vi "Get HSB.vi"(8 "error in (no error)":errorcluster caption="错误输入（无错误）", 11 "Color 输入":refnum<class "Color.lvclass"> caption="DNL_LabVIEW Object in") -> (0 "error out":errorcluster caption="错误输出", 2 "HSB":T1, 3 "Color 输出":refnum<class "Color.lvclass"> caption="DNL_LabVIEW Object out")   [LabVIEW 2012, in "Color.lvclass"]
uses:
  Color.lvclass
  HSB.ctl
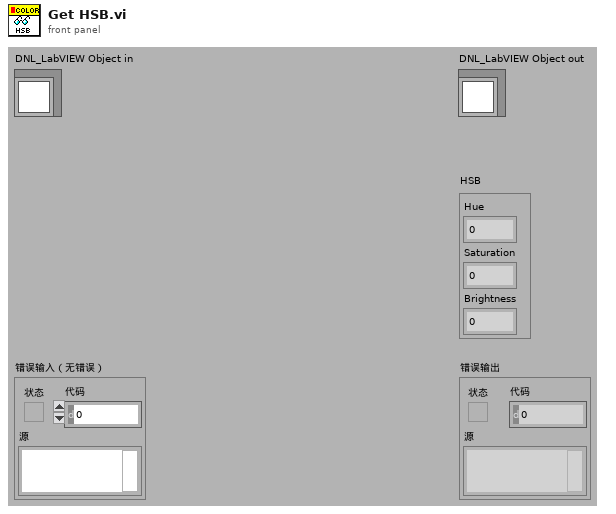
[diagram p1: front panel]
types:
  T1 = typedef "Color.lvclass/HSB.ctl" = cluster{"Hue":sgl, "Saturation":sgl, "Brightness":sgl}
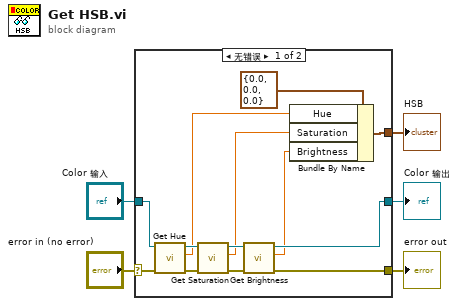
[diagram p0: block diagram]
diagram:
  n1 = case shown="无错误" "error in (no error)" {
    selector: "error in (no error)" -> [w15 w20]
    tunnel: [w6 w20] -> w4
    tunnel: [w12 w19] -> w2
    tunnel: "Color 输入" -> [w18 w19]
    tunnel: [w8 _] -> w1
    frame No Error {
      n2 = call "Get Hue.vi"("error in (no error)"=w15, "Color 输入"=w18) -> ("error out"=w14:errorcluster, "GetHue"=w11:sgl, "Color 输出"=w17:refnum<class "Color.lvclass">)  [unwired: 7 in]
      n3 = call "Get Saturation.vi"("error in (no error)"=w14, "Color 输入"=w17) -> ("error out"=w13:errorcluster, "GetSaturation"=w10:sgl, "Color 输出"=w16:refnum<class "Color.lvclass">)  [unwired: 7 in]
      n4 = call "Get Brightness.vi"("error in (no error)"=w13, "Color 输入"=w16) -> ("error out"=w6:errorcluster, "GetBrightness"=w9:sgl, "Color 输出"=w12:refnum<class "Color.lvclass">)  [unwired: 7 in]
      n5 = Bundle By Name(cluster=T1 {"Hue"=0.0, "Saturation"=0.0, "Brightness"=0.0} ("HSB"), "Hue"=w11, "Saturation"=w10, "Brightness"=w9) -> (w8:T1)
    }
    frame Error {
    }
  }
  "error out" <- w4
  "Color 输出" <- w2
  "HSB" <- w1
